vi "Measure Current.vi"(8 "error in (no error)":errorcluster, 11 "2230G in":refnum<class "2230G.lvclass">) -> (0 "error out":errorcluster, 2 "Current":dbl, 3 "2230G out":refnum<class "2230G.lvclass">)   [LabVIEW 2018, in "2230G.lvlib" / "2230G.lvclass"]
uses:
  2230G.lvclass
  PPLs/Power Supply/Parent/Power_Supply.lvlibp/Power Supply.lvclass
  <instrlib>/Keithley KE22xx Series/Keithley KE22xx Series.lvlib
  C:/Projects/LabVIEW/PPLs/Power Supply/Parent/Power_Supply.lvlibp/Power Supply.lvclass
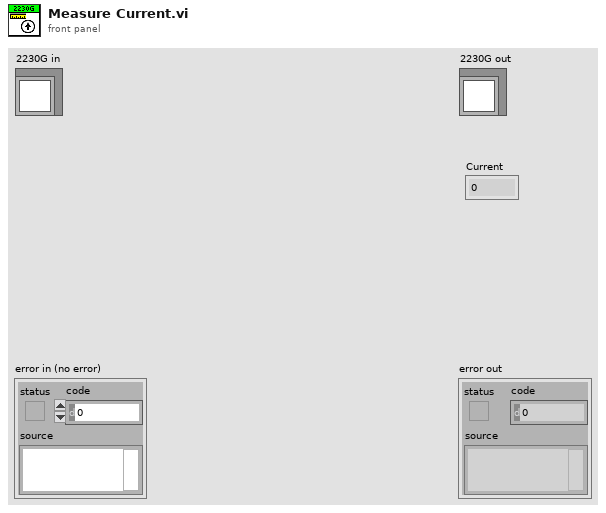
[diagram p1: front panel]
types:
  T1 = typedef "Power_Supply.lvlibp/Channel List.ctl" = enum16{"Channel 1", "Channel 2", "Channel 3", "Channel 4"}
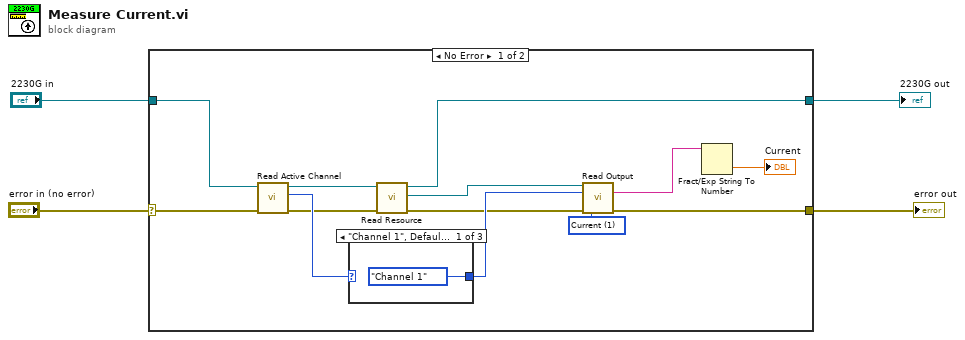
[diagram p0: block diagram]
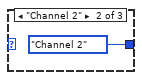
[diagram p2: hidden frame]
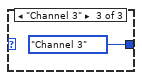
[diagram p3: hidden frame]
diagram:
  n1 = case shown="No Error" "error in (no error)" {
    selector: "error in (no error)" -> [w17 w22]
    tunnel: [w5 w22] -> w1
    tunnel: [w9 w21] -> w2
    tunnel: "2230G in" -> [w16 w21]
    frame No Error {
      w10 = u16 1 items=["Voltage", "Current", "Power"] ("Measurement Function (0:Voltage)")
      n2 = call "Read Active Channel.vi"("error in (no error)"=w17, "Power Supply in"=w16) -> ("error out"=w11:errorcluster, "Active Channel"=w13:T1, "Power Supply out"=w15:refnum<class "2230G.lvclass">)  [unwired: 7 in]
      n3 = case shown="\"Channel 1\", Default" w13 {
        tunnel: [enum16{"Channel 1", "Channel 2", "Channel 3"}."Channel 1" ("Channel Select") enum16{"Channel 1", "Channel 2", "Channel 3"}."Channel 2" ("Channel Select") enum16{"Channel 1", "Channel 2", "Channel 3"}."Channel 3" ("Channel Select")] -> w12
        frame "Channel 1", Default {
        }
        frame "Channel 2" {
        }
        frame "Channel 3" {
        }
      }
      n4 = call "Read Resource.vi"("error in"=w11, "Power Supply in"=w15) -> ("error out"=w6:errorcluster, "Resource"=w14:refnum<visa-resource-name>, "Power Supply out"=w9:refnum<class "2230G.lvclass">)  [unwired: 7 in]
      n5 = call <instrlib>:"Read Output.vi"("VISA resource name"=w14, "Channel Select"=w12, "Measurement Function (0:Voltage)"=w10, "error in (no error)"=w6) -> ("Measurement"=w8:string, "error out"=w5:errorcluster)  [unwired: 9 in, 1 out]
      n6 = Fract/Exp String To Number(string=w8) -> (number=→"Current":dbl)  [unwired: 3 in, 1 out]
    }
    frame Error {
    }
  }
  "error out" <- w1
  "2230G out" <- w2
